vi "2.2 Steering Chooser.vi"() -> ()   [LabVIEW 2011]
doc: "Takes waypoint and boat location information from the global variable and places the approproate rudder position command on the global.\nFor Drive waypoints, this VI simply tries to make the boat's heading the same as the heading between the boat and the waypoint. TODO: this does not account for drift -- it assumes that the boat will go where it is pointed which is not always the case.\n\nTODO: important: As of 11/17 this VI only works for the Drive option.\nTODO: ideally this VI would run on any update of the boat location or waypoint location, and not otherwise."
uses:
  2 Typedefs/heading.ctl
  2x3-RIO-OCU Comm/2x3 Typedefs/ocuWaypoint.ctl
  2x3-RIO-OCU Comm/2x3 Typedefs/waypointTypes.ctl
  2 Typedefs/UTM Location.ctl
  2 Typedefs/Velocity.ctl
  2 Globals/2 Global.vi
panel:
  in  "maximum rudder deflection":T1=-30.0 format="%05.1f"
  out "Robot\nHeading":T1 format="%05.1f"
  out "Angle to waypt":T1 format="%05.1f"
  out "Distance to Waypoint":T2
  out "Robot UTM Location":T3
  out "Waypoint":T4 {"Point Type" items=["Drive", "Round Port", "Round Starboard", "Stay"]}
  out "desired delta heading":T1 format="%05.1f"
  # "Steering Chooser simply turns the rudder to aim the boat's bow towards the next waypoint.\n\nTODO: currently only implements Drive waypoints. Also this is extremely stupid.\nImplement avoidance, stay-in-area, and maybe a PID loop."
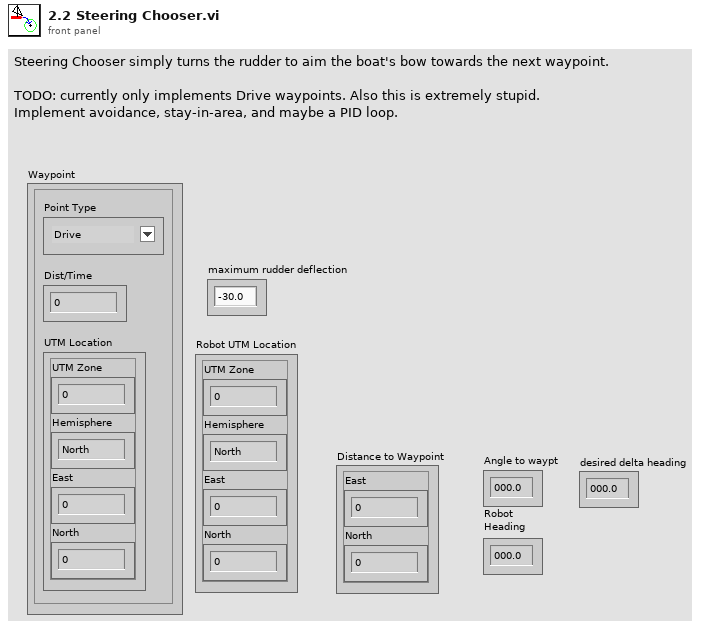
[diagram p1: front panel]
types:
  T1 = typedef "heading.ctl" = dbl
  T2 = typedef "Velocity.ctl" = cluster{"East":dbl, "North":dbl}
  T3 = typedef "UTM Location.ctl" = cluster{"UTM Zone":dbl, "Hemisphere":enum16{"North", "South"}, "East":dbl, "North":dbl}
  T4 = typedef "ocuWaypoint.ctl" = cluster{"Point Type":T5, "Dist/Time":dbl, "UTM Location":T3}
  T5 = typedef "waypointTypes.ctl" = u16
  T6 = typedef "ocuWaypoints.ctl" = cluster{"Waypoints Array":T4[], "Current Waypoint":dbl}
  T7 = cluster{"UTM Zone":dbl, "Hemisphere":u16, "East":dbl, "North":dbl}
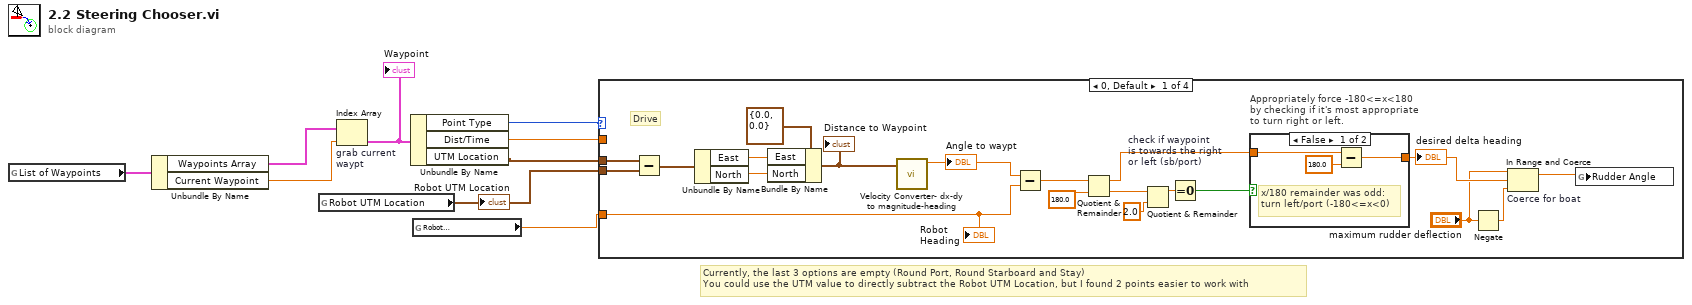
[diagram p0: block diagram]
diagram:
  # "Currently, the last 3 options are empty (Round Port, Round Starboard and Stay)\nYou could use the UTM value to directly subtract the Robot UTM Location, but I found 2 points easier to work with"
  n1 = global read "2 Global.vi" "List of Waypoints"() -> (w7:T6)
  n2 = Unbundle By Name(w7) -> ("Waypoints Array"=w9:T4[], "Current Waypoint"=w8:dbl)
  n3 = global read "2 Global.vi" "Robot UTM Location"() -> (w6:T3)
  "Robot UTM Location" <- w6
  n4 = Index Array "grab current\nwaypt"(array=w9, index=w8) -> (element=w4:T4)
  "Waypoint" <- w4
  n5 = Unbundle By Name(w4) -> ("Point Type"=w1:T5, "Dist/Time"=w2:dbl, "UTM Location"=w3:T3)
  n6 = global read "2 Global.vi" "Robot\nHeading"() -> (w5:T1)
  n7 = case shown="0, Default" w1 {
    tunnel: w3 -> [w29 _ _ _]
    tunnel: w6 -> [w28 _ _ _]
    tunnel: w5 -> [w22 _ _ _]
    tunnel: w2 -> [_ _ _ _]
    frame 0, Default {
      # "Drive"
      n8 = Subtract(x=w29, y=w28) -> (x-y=w27:T7)
      n9 = Unbundle By Name(w27) -> ("East"=w26:dbl, "North"=w25:dbl)
      n10 = Bundle By Name(cluster=T2 {"East"=0.0, "North"=0.0} ("Vector In"), "East"=w26, "North"=w25) -> (w23:T2)
      "Distance to Waypoint" <- w23
      n11 = call "Velocity Converter- dx-dy to magnitude-heading.vi"("Vector In"=w23) -> ("Heading Out"=w20:T1)  [unwired: 9 in, 1 out]
      "Angle to waypt" <- w20
      n12 = Subtract(x=w20, y=w22) -> (x-y=w18:T1)
      n13 = Quotient & Remainder ("shift to -180<x<180")(x=w18, y=T1 180.0) -> (x-y*floor(x/y)=w13:T1, floor(x/y)=w17:T1)
      n14 = Quotient & Remainder ("shift to -180<x<180")(x=w17, y=T1 2.0) -> (x-y*floor(x/y)=w15:T1)  [unwired: 1 out]
      n15 = Equal To 0? "check if waypoint\nis towards the right\nor left (sb/port)"(x=w15) -> (x = 0?=w14:bool)
      n16 = case "Appropriately force -180<=x<180\nby checking if it's most appropriate\nto turn right or left." shown="False" w14 {
        tunnel: w13 -> [w31 w33]
        tunnel: [w30 w33] -> w12
        frame False {
          # "x/180 remainder was odd:\nturn left/port (-180<=x<0)"
          n17 = Subtract(x=w31, y=T1 180.0) -> (x-y=w30:T1)
        }
        frame True {
          # "x/180 remainder was\neven: turn right/sb\n(0<=x<180)"
        }
      }
      "desired delta heading" <- w12
      n18 = Negate(x="maximum rudder deflection") -> (-x=w10:T1)
      n19 = In Range and Coerce "Coerce for boat"(upper limit="maximum rudder deflection", x=w12, lower limit=w10) -> (coerced(x)=w21:T1)  [unwired: 1 out]
      n20 = global write "2 Global.vi" "Rudder Angle"(w21) -> ()
      "Robot\nHeading" <- w22
    }
    frame 1 {
      # "Round Port"
    }
    frame 2 {
      # "Round Starboard"
    }
    frame 3 {
      # "Stay"
    }
  }
